vi "test_Set Instrument Addon Name.vi"(8 "error in (no error)":errorcluster, 11 "TestCase in":refnum<class "Instrument Addon Scripting API Custom Device Unit Tests.lvclass">) -> (0 "error out":errorcluster, 3 "TestCase out":refnum<class "Instrument Addon Scripting API Custom Device Unit Tests.lvclass">)   [LabVIEW 2019, in "Instrument Addon Scripting API Custom Device Unit Tests.lvclass"]
uses:
  Instrument Addon Scripting API Custom Device Unit Tests.lvclass
  Instrument Addon Scripting API Custom Device Unit Tests.lvclass/Instrument Addon Scripting API Custom Device Unit Tests.ctl
  <vilib>/addons/_JKI Toolkits/VI Tester/TestCase.llb/TestCase.lvclass
  APIs/Scripting API/Instrument Addon Scripting API.lvlib
  C:/Program Files (x86)/National Instruments/LabVIEW 2019/vi.lib/addons/_JKI Toolkits/VI Tester/TestCase.llb/TestCase.lvclass
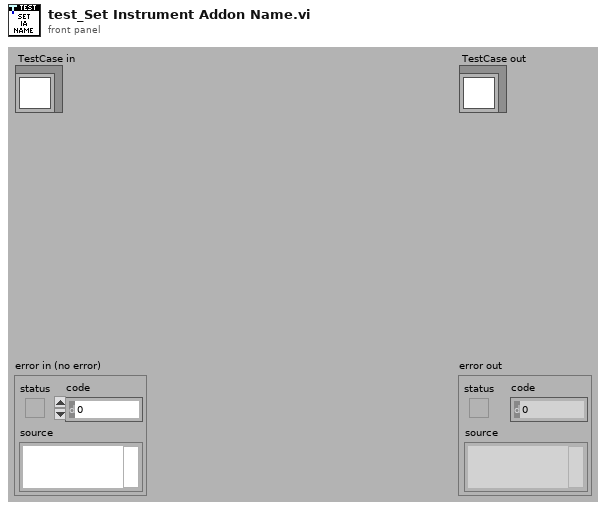
[diagram p1: front panel]
types:
  T1 = typedef "Custom Device API.lvlib/Custom Device Item Ref.ctl" = u64
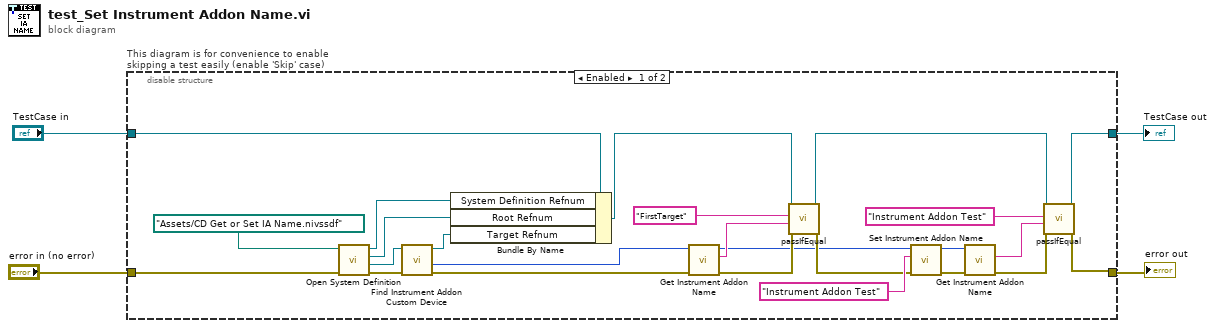
[diagram p0: block diagram]
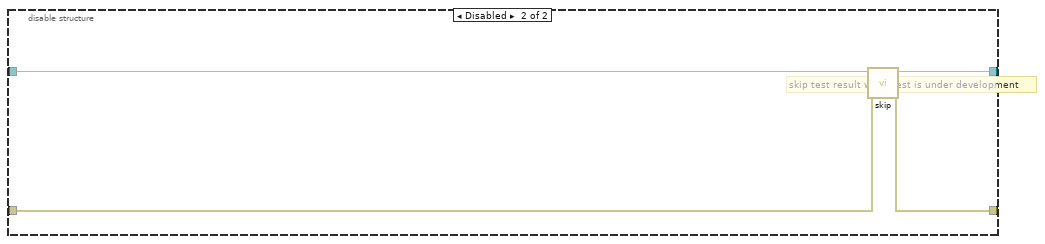
[diagram p2: hidden frame]
diagram:
  n1 = disable-structure "This diagram is for convenience to enable skipping a test easily (enable 'Skip' case)" shown="Enabled" {
    disable-tunnel: "TestCase in" -> [w9 w33]
    disable-tunnel: [w29 w31] -> w1
    disable-tunnel: [w28 w32] -> w3
    disable-tunnel: "error in (no error)" -> [w27 w30]
    frame Enabled {
      n2 = call "Open System Definition.vi"("error in (no error)"=w27, "System Definition File"=path "Assets/CD Get or Set IA Name.nivssdf") -> ("error out"=w26:errorcluster, "Target Refnum"=w25:refnum<k24>, "Root Refnum"=w6:refnum<k24>, "System Definition Refnum"=w7:refnum<k24>)  [unwired: 6 in]
      n3 = call "Find Instrument Addon Custom Device.vi"("error in"=w26, "target in"=w25) -> ("error out"=w22:errorcluster, "NodeID"=w16:u64, "target out"=w5:refnum<k24>)  [unwired: 7 in]
      n4 = Bundle By Name(cluster=w9, "System Definition Refnum"=w7, "Root Refnum"=w6, "Target Refnum"=w5) -> (w8:refnum<class "Instrument Addon Scripting API Custom Device Unit Tests.lvclass">)
      n5 = call "Get Instrument Addon Name.vi"("error in (no error)"=w22, "instrument addon refnum in"=w16) -> ("error out"=w15:errorcluster, "name"=w13:string, "instrument addon refnum out"=w11:T1)  [unwired: 7 in]
      n6 = call-dynamic "passIfEqual.vi"("error in (no error)"=w15, "y"=w13, "x"="FirstTarget" ("Name"), "TestCase in"=w8) -> ("error out"=w14:errorcluster, "TestCase out"=w10:refnum<class "Instrument Addon Scripting API Custom Device Unit Tests.lvclass">)  [unwired: 6 in]
      n7 = call "Set Instrument Addon Name.vi"("error in (no error)"=w14, "name"="Instrument Addon Test" ("Name"), "instrument addon refnum in"=w11) -> ("error out"=w21:errorcluster, "instrument addon refnum out"=w18:T1)  [unwired: 7 in]
      n8 = call "Get Instrument Addon Name.vi"("error in (no error)"=w21, "instrument addon refnum in"=w18) -> ("error out"=w20:errorcluster, "name"=w17:string)  [unwired: 7 in, 1 out]
      n9 = call-dynamic "passIfEqual.vi"("error in (no error)"=w20, "y"=w17, "x"="Instrument Addon Test", "TestCase in"=w10) -> ("error out"=w28:errorcluster, "TestCase out"=w29:refnum<class "Instrument Addon Scripting API Custom Device Unit Tests.lvclass">)  [unwired: 6 in]
    }
    frame Disabled {
      # "skip test result while test is under development"
      n10 = call <vilib>:"skip.vi"("error in (no error)"=w30, "TestCase in"=w33) -> ("error out"=w32:errorcluster, "TestCase out"=w31:refnum<class "Instrument Addon Scripting API Custom Device Unit Tests.lvclass">)  [unwired: 8 in]
    }
  }
  "error out" <- w3
  "TestCase out" <- w1
